vi "Stop Measure.vi"(8 "error in (no error)":errorcluster, 11 "Device ID (0)":i32) -> (0 "error out":errorcluster, 3 "Device ID out":i32)   [LabVIEW 2015, in "KEYENCE LJ-X8000A.lvlib"]
doc: "This function stops batch measurement. \nWhen batch measurement has not been started, nothing happens and there is no error."
uses:
  KEYENCE LJ-X8000A.lvlib
panel:
  # "(c) 2019 KEYENCE CORPORATION.  ALL RIGHTS RESERVED."
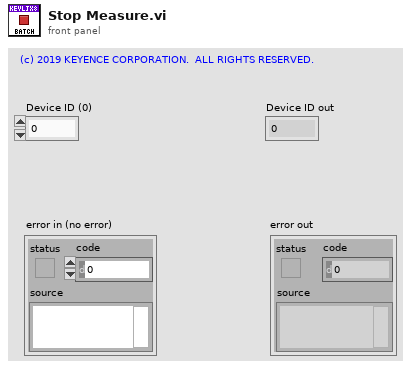
[diagram p1: front panel]
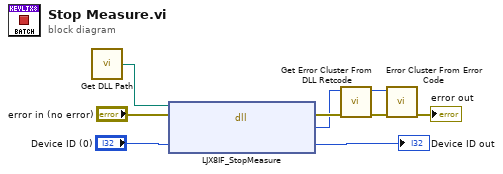
[diagram p0: block diagram]
diagram:
  n1 = call "Get DLL Path.vi"() -> ("DLL Path"=w6:path)  [unwired: 3 in]
  n2 = dll-call lib="C:/Program Files (x86)/National Instruments/LabVIEW 2018/instr.lib/KEYENCE LJ-X8000/LJX8_IF.*" fn="LJX8IF_StopMeasure"(path in=w6, error in="error in (no error)", "lDeviceId"="Device ID (0)") -> (error out=w4:errorcluster, "lRetCode"=w3:i32, "lDeviceId"=→"Device ID out":i32)  [unwired: 1 in, 1 out]
  n3 = call "Get Error Cluster From DLL Retcode.vi"("error in (no error)"=w4, "DLL Return Code"=w3) -> ("error out"=w5:errorcluster, "VI Error Code"=w1:i32)  [unwired: 8 in]
  n4 = call <vilib>:"Error Cluster From Error Code.vi"("error in (no error)"=w5, "error code (0)"=w1) -> ("error out"=→"error out":errorcluster)  [unwired: 7 in]
